vi "DC Motor Example2.vi"() -> ()   [LabVIEW 2015]
uses:
  <userlib>/KNR OS 3.0 LabVIEW Toolkit/Type Definition/Resource.ctl
  <userlib>/KNR OS 3.0 LabVIEW Toolkit/Type Definition/DC Motor Port.ctl
  <userlib>/KNR OS 3.0 LabVIEW Toolkit/General/KNR3 Open(Direct).vi
panel:
  in  "Reset 2":bool
  in  "Reverse? 2":bool
  out "Velocity (cts/sec) 2":dbl
  out "Position 2":i32
  in  "stop 2":bool
  in  "Port 2":T1=4 items=["DS1"=4, "DS2"=5, "DS3"=6, "DS4"=7]
  in  "Numeric":i32
  in  "Port":T1=4 items=["DS1"=4, "DS2"=5, "DS3"=6, "DS4"=7]
  in  "Resource":T2
  in  "stop":bool
  in  "Enable Motor":bool
  in  "Speed (+-100%)":dbl=50.0
  out "Position":i32
  out "Velocity (cts/sec)":dbl
  in  "Reverse?":bool
  in  "Reset":bool
  # "KNR/KNRm\nPort5=DS1\nPort6=DS2\nPort7=DS3\nPort8=DS4"
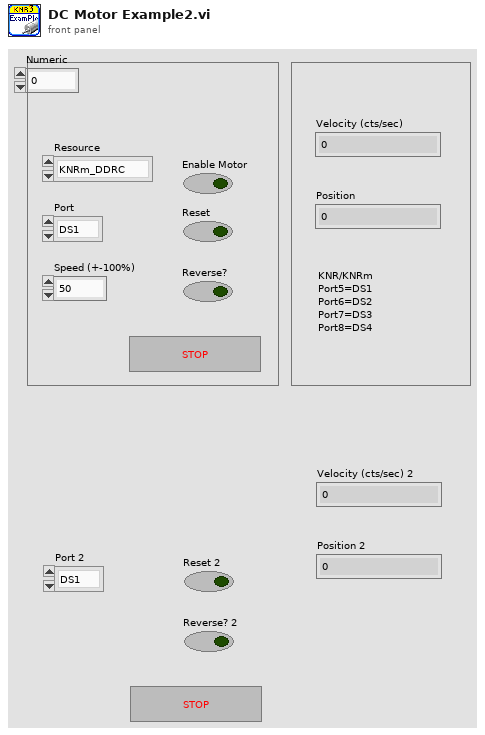
[diagram p1: front panel]
types:
  T1 = typedef "DC Motor Port.ctl" = u16
  T2 = typedef "Resource.ctl" = enum16{"KNRm_DDRC", "KNRm_DDDD", "KNRm_DDDR", "KNRm_DDDC", "KNR"}
  T3 = typedef "KNR3 Reference.ctl" = cluster{"FPGA Session":refnum<class "FPGA Interface Base.lvclass">, "Resource":T2}
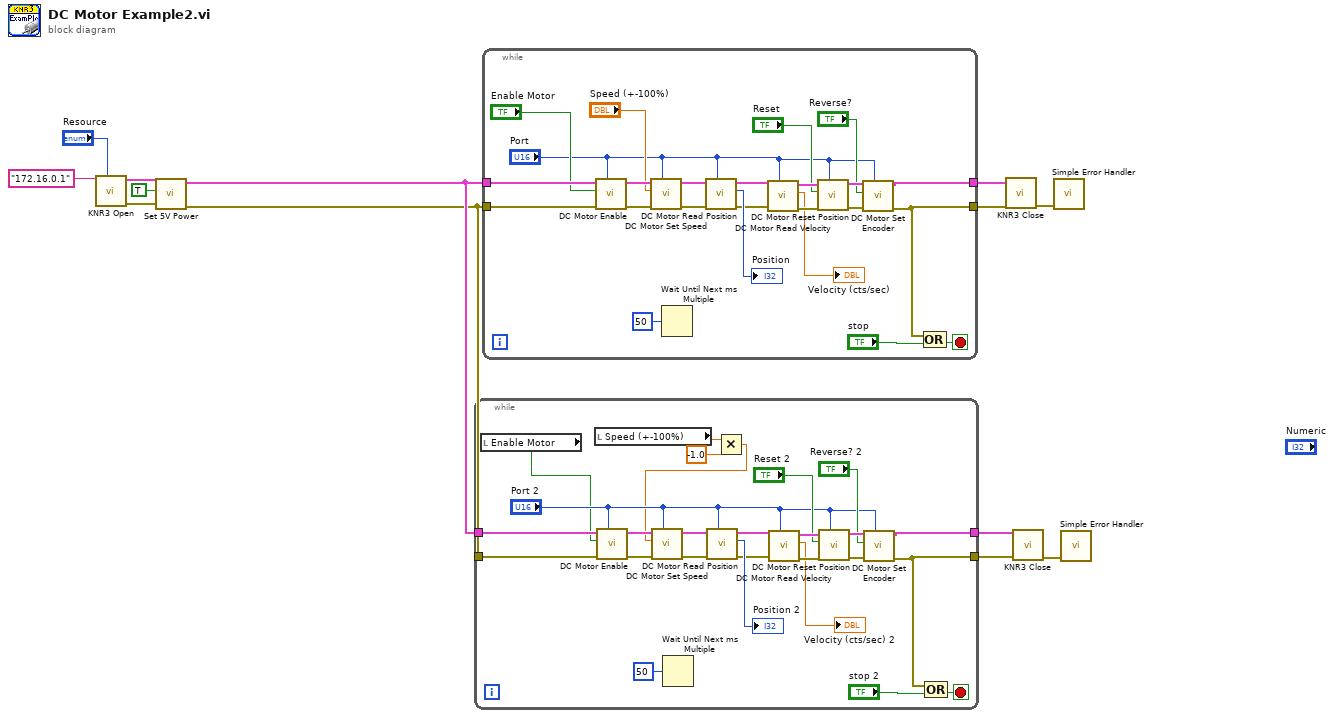
[diagram p0: block diagram]
diagram:
  n1 = call-poly <userlib>:"KNR3 Open.vi"("Resource"="Resource", "IP"="172.16.0.1") -> ("error out"=w7:errorcluster, "KNR out"=w9:T3)  [unwired: 8 in]
  n2 = call <userlib>:"Set 5V Power.vi"("error in (no error)"=w7, "5V Power(T)"=TRUE ("5V Power"), "KNR in"=w9) -> ("error out"=w1:errorcluster, "KNR out"=w2:T3)  [unwired: 7 in]
  n3 = while {
    tunnel: w2 -> [w39]
    tunnel: w1 -> [w35]
    tunnel: [w24] -> w3
    tunnel: [w25] -> w4
    stop <- w31 stop-if-true
    n4 = local read "Enable Motor"() -> (w17:bool)
    n5 = local read "Speed (+-100%)"() -> (w16:dbl)
    n6 = call <userlib>:"DC Motor Enable.vi"("Port (DS1)"="Port 2", "error in (no error)"=w35, "Enable Motor(F)"=w17, "KNR in"=w39) -> ("error out"=w34:errorcluster, "KNR out"=w38:T3)  [unwired: 6 in]
    n7 = Wait Until Next ms Multiple(millisecond multiple=u32 50) -> ()  [unwired: 1 out]
    n8 = Multiply(x=w16, y=-1.0) -> (x*y=w14:dbl)
    n9 = call <userlib>:"DC Motor Set Speed.vi"("Port (DS1)"="Port 2", "error in (no error)"=w34, "Speed (+-100%)"=w14, "KNR in"=w38) -> ("error out"=w33:errorcluster, "KNR out"=w37:T3)  [unwired: 6 in]
    n10 = call <userlib>:"DC Motor Read Position.vi"("Port (DS1)"="Port 2", "error in (no error)"=w33, "KNR in"=w37) -> ("error out"=w28:errorcluster, "Position"=→"Position 2":i32, "KNR out"=w29:T3)  [unwired: 6 in]
    n11 = call <userlib>:"DC Motor Read Velocity.vi"("Port (DS1)"="Port 2", "error in (no error)"=w28, "KNR in"=w29) -> ("error out"=w22:errorcluster, "Velocity (cts/sec)"=→"Velocity (cts/sec) 2":dbl, "KNR out"=w27:T3)  [unwired: 6 in]
    n12 = call <userlib>:"DC Motor Reset Position.vi"("Port (DS1)"="Port 2", "error in (no error)"=w22, "Reset(F)"="Reset 2", "KNR in"=w27) -> ("error out"=w23:errorcluster, "KNR out"=w26:T3)  [unwired: 6 in]
    n13 = call <userlib>:"DC Motor Set Encoder.vi"("Port (DS1)"="Port 2", "error in (no error)"=w23, "Reverse?(F)"="Reverse? 2", "KNR in"=w26) -> ("error out"=w24:errorcluster, "KNR out"=w25:T3)  [unwired: 6 in]
    n14 = Compound Arithmetic op=OR(w24, "stop 2") -> (w31:bool)
  }
  n15 = while {
    tunnel: w2 -> [w63]
    tunnel: w1 -> [w57]
    tunnel: [w46] -> w11
    tunnel: [w47] -> w12
    stop <- w53 stop-if-true
    n16 = call <userlib>:"DC Motor Enable.vi"("Port (DS1)"="Port", "error in (no error)"=w57, "Enable Motor(F)"="Enable Motor", "KNR in"=w63) -> ("error out"=w56:errorcluster, "KNR out"=w62:T3)  [unwired: 6 in]
    n17 = call <userlib>:"DC Motor Set Speed.vi"("Port (DS1)"="Port", "error in (no error)"=w56, "Speed (+-100%)"="Speed (+-100%)", "KNR in"=w62) -> ("error out"=w55:errorcluster, "KNR out"=w61:T3)  [unwired: 6 in]
    n18 = Wait Until Next ms Multiple(millisecond multiple=u32 50) -> ()  [unwired: 1 out]
    n19 = call <userlib>:"DC Motor Read Position.vi"("Port (DS1)"="Port", "error in (no error)"=w55, "KNR in"=w61) -> ("error out"=w50:errorcluster, "Position"=→"Position":i32, "KNR out"=w51:T3)  [unwired: 6 in]
    n20 = call <userlib>:"DC Motor Read Velocity.vi"("Port (DS1)"="Port", "error in (no error)"=w50, "KNR in"=w51) -> ("error out"=w44:errorcluster, "Velocity (cts/sec)"=→"Velocity (cts/sec)":dbl, "KNR out"=w49:T3)  [unwired: 6 in]
    n21 = call <userlib>:"DC Motor Reset Position.vi"("Port (DS1)"="Port", "error in (no error)"=w44, "Reset(F)"="Reset", "KNR in"=w49) -> ("error out"=w45:errorcluster, "KNR out"=w48:T3)  [unwired: 6 in]
    n22 = call <userlib>:"DC Motor Set Encoder.vi"("Port (DS1)"="Port", "error in (no error)"=w45, "Reverse?(F)"="Reverse?", "KNR in"=w48) -> ("error out"=w46:errorcluster, "KNR out"=w47:T3)  [unwired: 6 in]
    n23 = Compound Arithmetic op=OR(w46, "stop") -> (w53:bool)
  }
  n24 = call <userlib>:"KNR3 Close.vi"("error in (no error)"=w11, "KNR in"=w12) -> ("error out"=w10:errorcluster)  [unwired: 9 in]
  n25 = call <userlib>:"KNR3 Close.vi"("error in (no error)"=w3, "KNR in"=w4) -> ("error out"=w5:errorcluster)  [unwired: 9 in]
  n26 = call <vilib>:"Simple Error Handler.vi"("error in (no error)"=w10) -> ()  [unwired: 4 in, 5 out]
  n27 = call <vilib>:"Simple Error Handler.vi"("error in (no error)"=w5) -> ()  [unwired: 4 in, 5 out]
